vi "Hood Jog.vi"(7 "Description":string, 8 "Command Info In":T1, 10 "Limelight? (F)":bool, 11 "Setpoint":dbl) -> (0 "Command Info Out":T1)   [LabVIEW 2019]
doc: "This template is useful for immediate subsystem actions that do not need deadband filtering\n\nBe sure to right-click and select New from Template and save with a new command name."
uses:
  <vilib>/Rock Robotics/WPI/Framework/Command Status Info.ctl
  <vilib>/Rock Robotics/WPI/Framework/Completion Status.ctl
  <vilib>/Rock Robotics/WPI/Framework/Completion Notifier.ctl
  Implementation/Hood Setpoints.ctl
  Implementation/Hood Operations.ctl
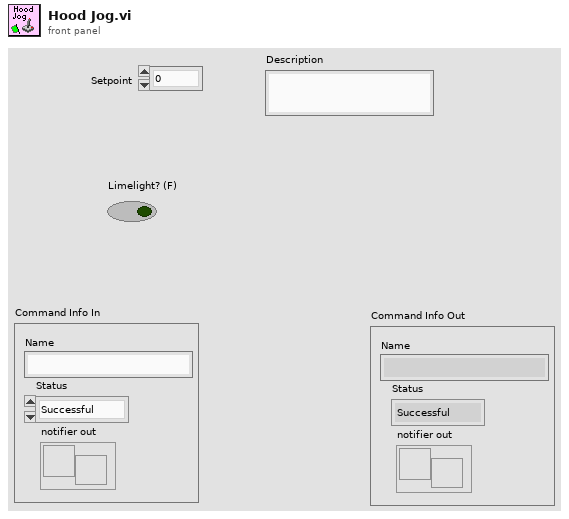
[diagram p1: front panel]
types:
  T1 = typedef "Command Status Info.ctl" = cluster{"Name":string, "Status":T2, "notifier out":T3}
  T2 = typedef "Completion Status.ctl" = enum16{"Successful", "Aborted", "Incomplete"}
  T3 = typedef "Completion Notifier.ctl" = refnum<notifier>
  T4 = typedef "Hood Setpoints.ctl" = cluster{"Operation":T5, "Setpoint":dbl, "Duration":dbl}
  T5 = typedef "Hood Operations.ctl" = enum16{"Reserve", "Read Current", "Immediate", "Jog", "Hood Setpoint", "Hood Stow", "Hood Restore", "Hood Change Saved Setpoint", "Hood Limelight"}
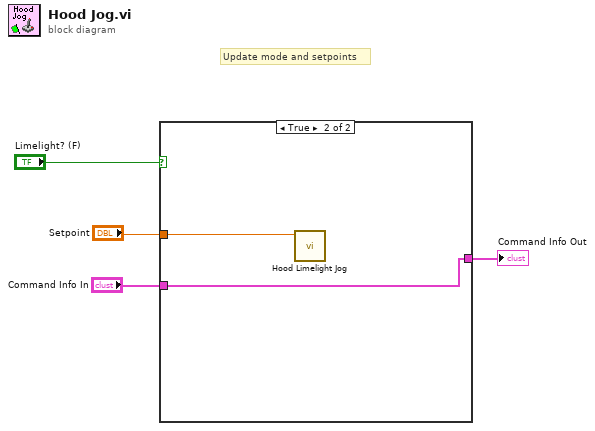
[diagram p0: block diagram]
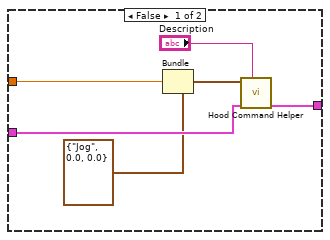
[diagram p2: hidden frame]
diagram:
  # "Update mode and setpoints"
  n1 = case shown="True" "Limelight? (F)" {
    tunnel: [w10 w12] -> w4
    tunnel: "Command Info In" -> [w9 w12]
    tunnel: "Setpoint" -> [w6 w11]
    frame False {
      n2 = Bundle(cluster=T4 {"Operation"=enum."Jog", "Setpoint"=0.0, "Duration"=0.0} ("SubSystem Data"), "Setpoint"=w6) -> (w5:T4)  [unwired: 2 in]
      n3 = call "Hood Command Helper.vi"("Description"="Description", "Command Info In"=w9, "SubSystem Data"=w5) -> ("Command Info Out"=w10:T1)  [unwired: 6 in, 2 out]
    }
    frame True {
      n4 = call "Hood Limelight Jog.vi"("Jog Amount"=w11) -> ()  [unwired: 11 in]
    }
  }
  "Command Info Out" <- w4
